vi "get next data.vi"(1 "Monitor Data":bool, 2 "data interval (s)":i32) -> (0 "get next":bool)   [LabVIEW 2010]
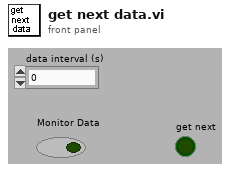
[diagram p1: front panel]
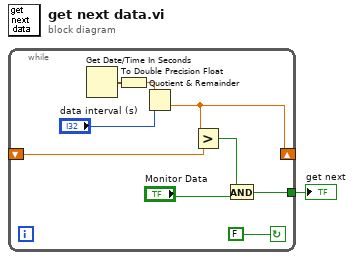
[diagram p0: block diagram]
diagram:
  n1 = while {
    tunnel: [w3] -> w1
    shift-left: _ -> [w7]
    shift-right: [w8] -> _
    stop <- FALSE continue-if-true
    n2 = Get Date/Time In Seconds() -> (seconds since 1Jan1904=w2:timestamp)
    n3 = To Double Precision Float(number=w2) -> (double precision float=w9:dbl)
    n4 = Quotient & Remainder(x=w9, y="data interval (s)") -> (floor(x/y)=w8:dbl)  [unwired: 1 out]
    n5 = Greater?(x=w8, y=w7) -> (0:w5:bool)
    n6 = And(x=w5, y="Monitor Data") -> (x .and. y?=w3:bool)
  }
  "get next" <- w1
